vi "Sync - Set Sessions.vi"(0 "TSM context":T1, 5 "Instrument Name":string, 7 "Channel Group  Id":string, 9 "Sync Session":refnum<k15>, 11 "error in":errorcluster) -> (4 "TSM context out":T1, 15 "error out":errorcluster)   [LabVIEW 2020]
doc: "Associates an NI-Sync session with an NI-Sync Instrument Name."
uses:
  <vilib>/NI_TestStand_SemiconductorModule/NI_TestStand_Semiconductor_Module.lvlibp/PinMap/General/SemiconductorModuleContext.ctl
  <vilib>/NI_TestStand_SemiconductorModule/NI_TestStand_Semiconductor_Module.lvlibp
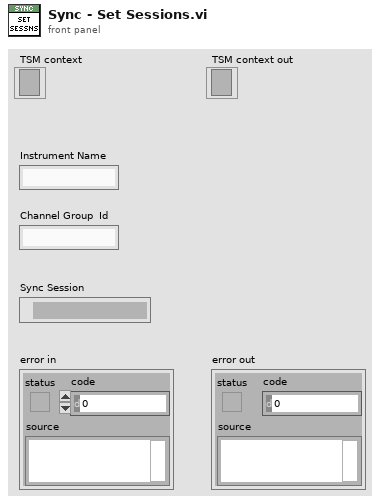
[diagram p1: front panel]
types:
  T1 = typedef "NI_TestStand_Semiconductor_Module.lvlibp/SemiconductorModuleContext.ctl" = refnum<k7>
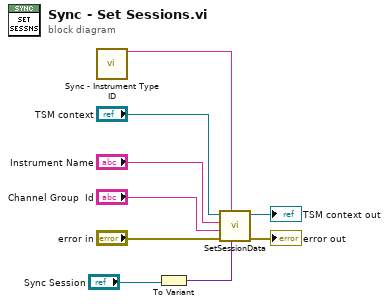
[diagram p0: block diagram]
diagram:
  n1 = call "Sync - Instrument Type ID.vi"() -> ("Instrument Type ID"=w2:string)  [unwired: 15 in]
  n2 = To Variant(anything="Sync Session") -> (Variant=w4:variant)
  n3 = call <vilib>:"SetSessionData.vi"("Session Data"=w4, "Instrument Type Id"=w2, "error in (no error)"="error in", "Channel Group Id"="Channel Group  Id", "Instrument Name"="Instrument Name", "Semiconductor Module Context"="TSM context") -> ("error out"=→"error out":errorcluster, "Semiconductor Module Context Out"=→"TSM context out":T1)  [unwired: 4 in]
